vi "GyroCounterIncrementor.vi"(11 "CurrentCounter":u8) -> (3 "NewCounter":u8)   [LabVIEW 2016, in "FPGAMockGyro.lvlib"]
uses:
  FPGAMockGyro.lvlib
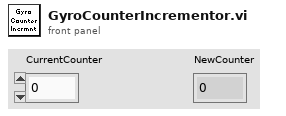
[diagram p1: front panel]
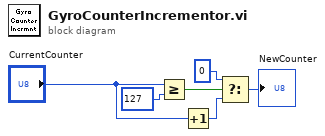
[diagram p0: block diagram]
diagram:
  n1 = Greater Or Equal?(x="CurrentCounter", y=u8 127) -> (x >= y?=w4:bool)
  n2 = Increment(x="CurrentCounter") -> (x+1=w6:u8)
  n3 = Select(t=u8 0, s=w4, f=w6) -> (s? t:f=→"NewCounter":u8)
